vi "GetDigitalPodSkew.vi"(3 "error in (no error)":errorcluster, 4 "Return Parameter":u8(ring) items=["Value", "Minimum", "Maximum"], 5 "Digital Pod (0: Digital Pod A)":u16(ring) items=["Pod A", "Pod B", "Pod C", "Pod D"], 6 "VISA resource name":refnum<visa-resource-name>) -> (0 "error out":errorcluster, 1 "Skew (s)":dbl format="%#_16g", 2 "VISA resource name out":refnum<visa-resource-name>)   [LabVIEW 2020, in "Active Technologies AWG3000.lvlib"]
uses:
  Active Technologies AWG3000.lvlib
panel:
  out "read buffer":string
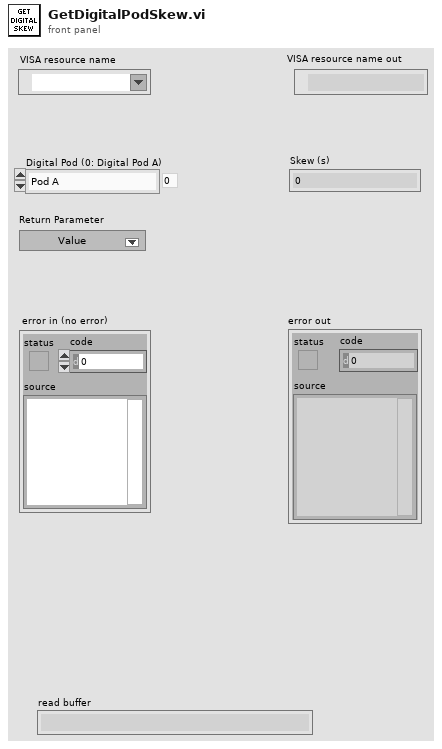
[diagram p1: front panel]
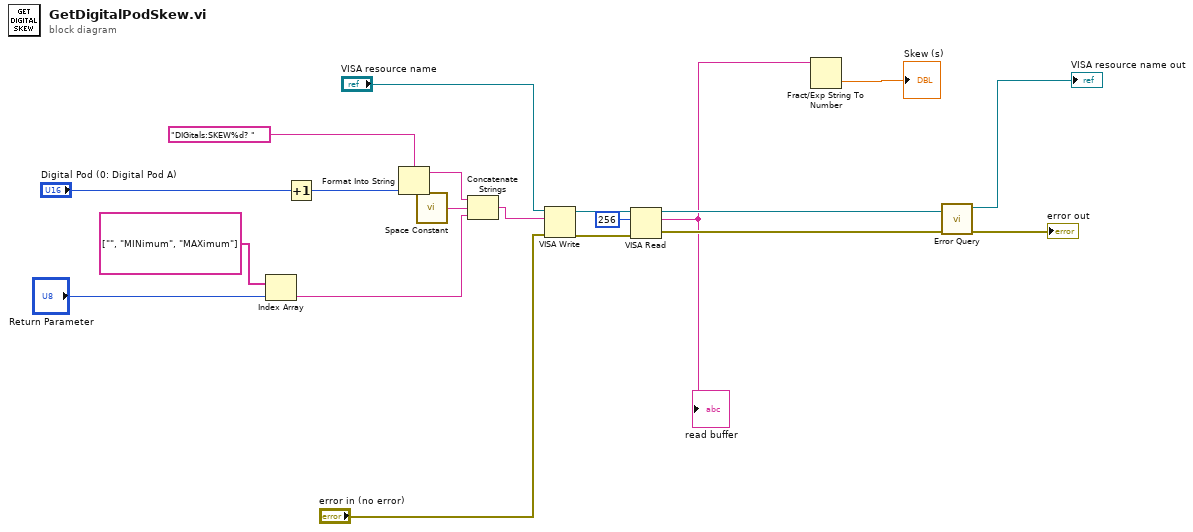
[diagram p0: block diagram]
diagram:
  n1 = Index Array(array=string[] ["", "MINimum", "MAXimum"], index="Return Parameter") -> (element=w5:string)
  n2 = Increment(x="Digital Pod (0: Digital Pod A)") -> (x+1=w17:u16)
  n3 = Format Into String(format string="DIGitals:SKEW%d? " ("write buffer"), w17) -> (resulting string=w14:string)  [unwired: 2 in, 1 out]
  n4 = call <vilib>:"Space Constant.vi"() -> ("String"=w4:string)
  n5 = Concatenate Strings(w14, w4, w5) -> (w13:string)
  n6 = VISA Write(VISA resource name="VISA resource name", write buffer=w13, error in (no error)="error in (no error)") -> (VISA resource name out=w12:refnum<visa-resource-name>, error out=w11:errorcluster)  [unwired: 1 out]
  n7 = VISA Read(VISA resource name=w12, byte count=u32 256, error in (no error)=w11) -> (VISA resource name out=w9:refnum<visa-resource-name>, read buffer=w2:string, error out=w8:errorcluster)  [unwired: 1 out]
  "read buffer" <- w2
  n8 = Fract/Exp String To Number(string=w2) -> (number=→"Skew (s)":dbl)  [unwired: 3 in, 1 out]
  n9 = call "Error Query.vi"("error in (no error)"=w8, "VISA resource name"=w9) -> ("error out"=→"error out":errorcluster, "VISA resource name out"=→"VISA resource name out":refnum<visa-resource-name>)  [unwired: 6 in, 2 out]
